vi "IKA_Eurostar60_Setup.vi"(7 "Checkbox":bool=TRUE, 8 "error in":errorcluster, 11 "COMMS":T1={"IKA_Eurostar"="COM1", "IKA"=FALSE, "Agilent"="COM1", "AGL"=FALSE}) -> (0 "error out":errorcluster)   [LabVIEW 2017]
uses:
  CRISTALIZADOR_COMM.ctl
  IKA_Eurostar60.ctl
panel:
  out "RUN":bool
  out "Par":dbl(knob) caption="Gauge" scale=0.0..10.0
  in  "Power On Button":bool
  out "PAR":dbl
  out "VELOCIDAD":dbl
  out "Velocidad":dbl(knob) caption="Gauge" scale=0.0..10.0
  out "Velocidad":dbl
  out "SETPOINT":dbl
  in  "Speed Button":bool
  in  "Giro Button":bool
  in  "Stop Button":bool
  in  "Start Button":bool
  # "Configuración rotador IKA.Euro60"
  # "asslcdms Feb2023 LV17"
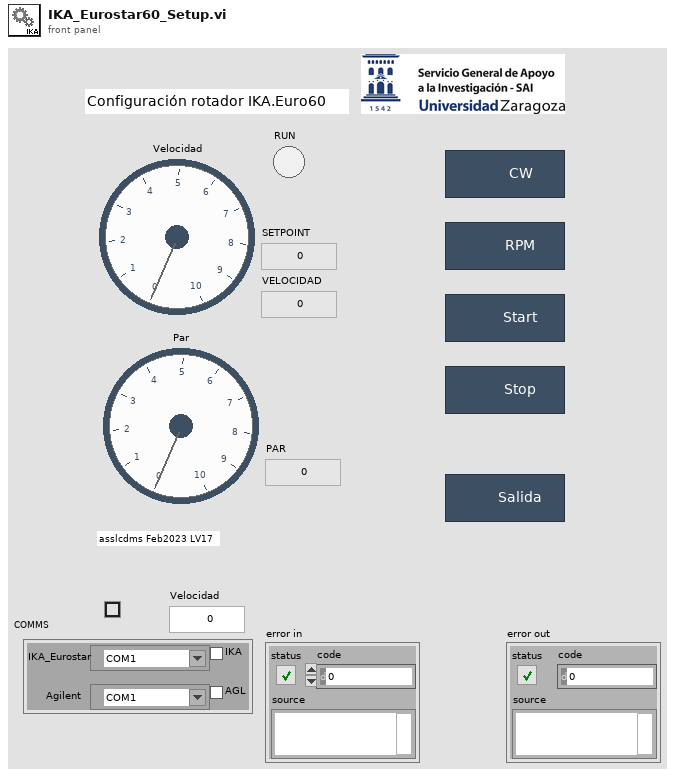
[diagram p1: front panel]
types:
  T1 = typedef "CRISTALIZADOR_COMM.ctl" = cluster{"IKA_Eurostar":refnum<visa-resource-name>, "IKA":bool, "Agilent":refnum<visa-resource-name>, "AGL":bool}
  T2 = typedef "IKA_Eurostar60.ctl" = enum16{"INICIALIZAR", "READ NOMBRE APARATO", "READ VALOR PT100", "READ VELOCIDAD ACTUAL", "READ PAR DE GIRO ACTUAL", "READ VELOCIDAD NOMINAL", "READ LIMITE PAR DE GIRO", "READ LIMITE VELOCIDAD", "READ VELOCIDAD SEGURIDAD", "SET VELOCIDAD NOMINAL", "SET LIMITE PAR DE GIRO", "SET LIMITE VELOCIDAD", "SET VELOCIDAD SEGURIDAD", "ARRANCAR MOTOR", "DETENER MOTOR", "RESET", "SET SENTIDO DE GIRO", "READ SENTIDO DE GIRO", "FINALIZAR"}
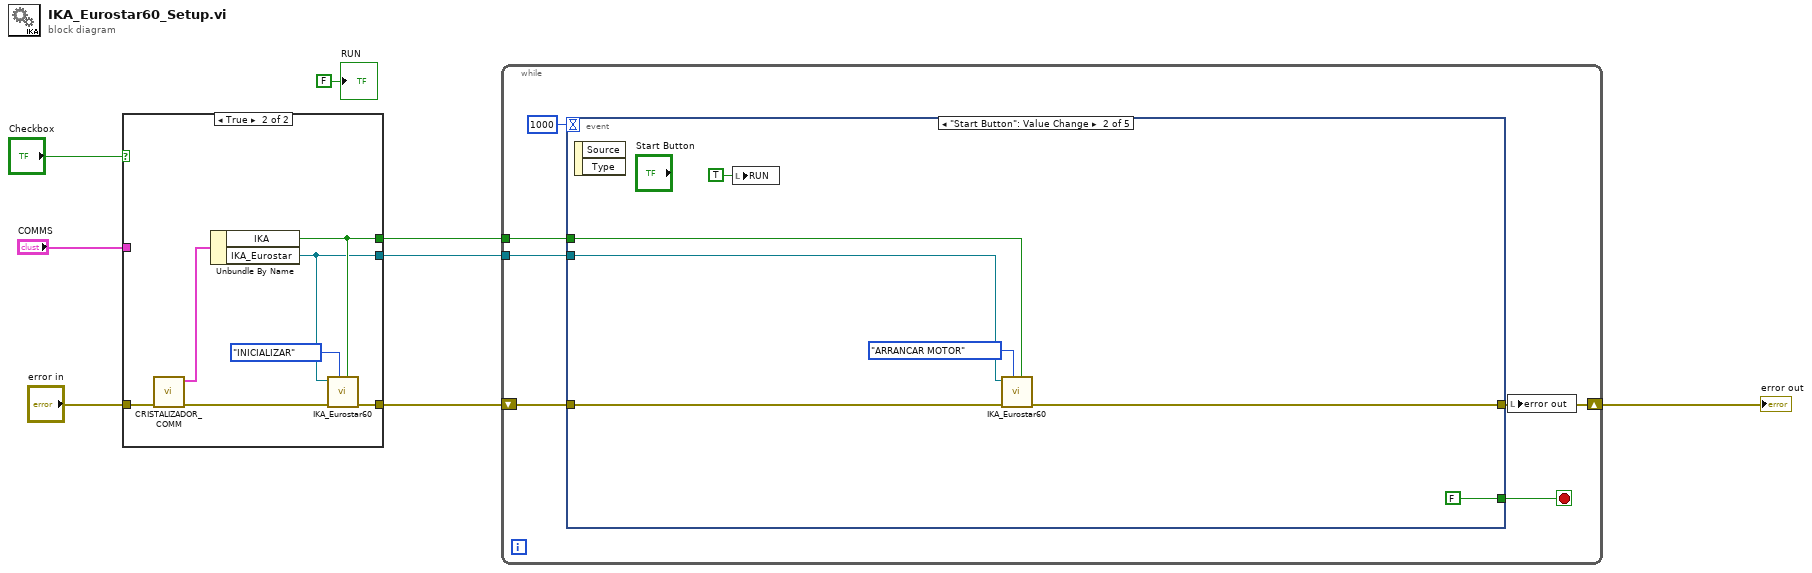
[diagram p0: block diagram]
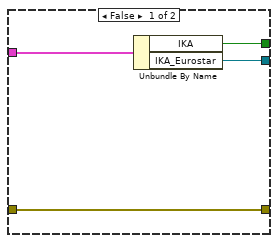
[diagram p2: hidden frame]
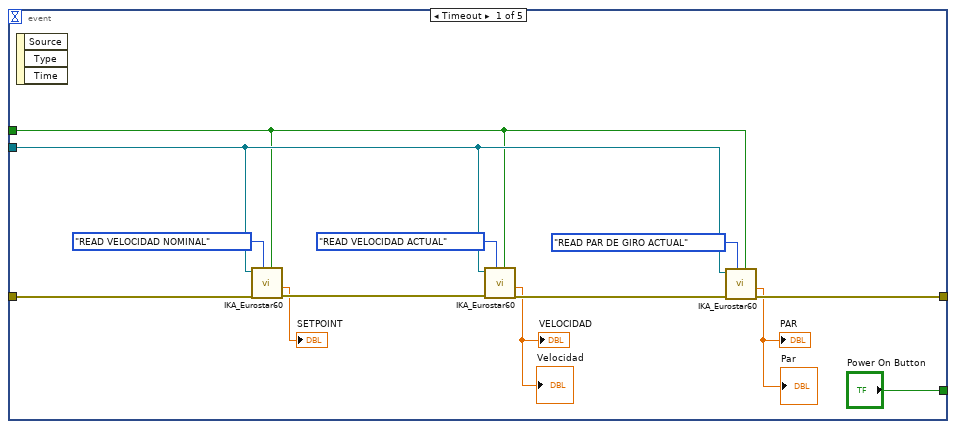
[diagram p3: hidden frame]
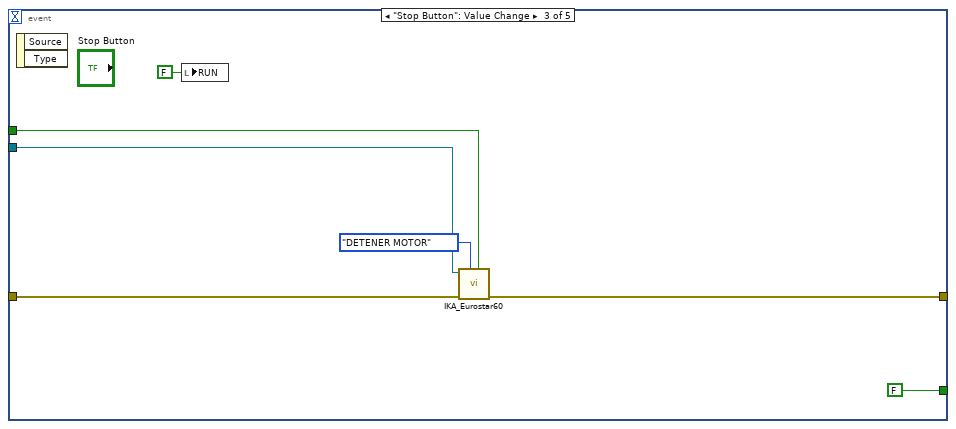
[diagram p4: hidden frame]
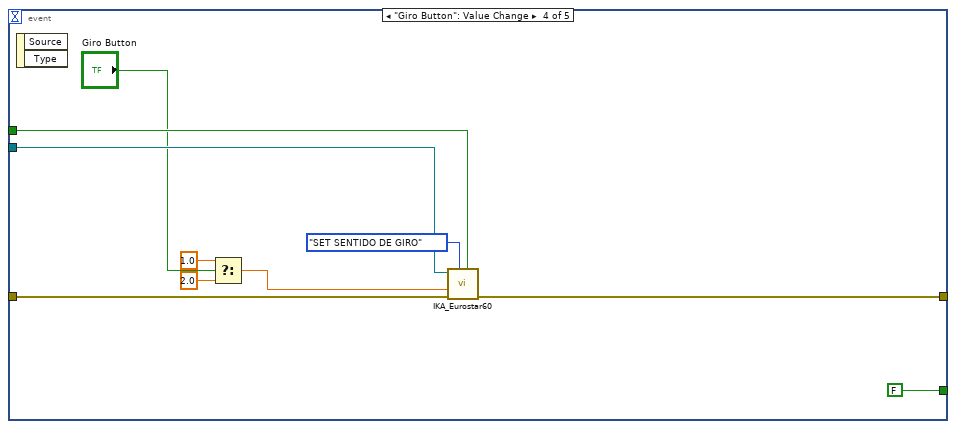
[diagram p5: hidden frame]
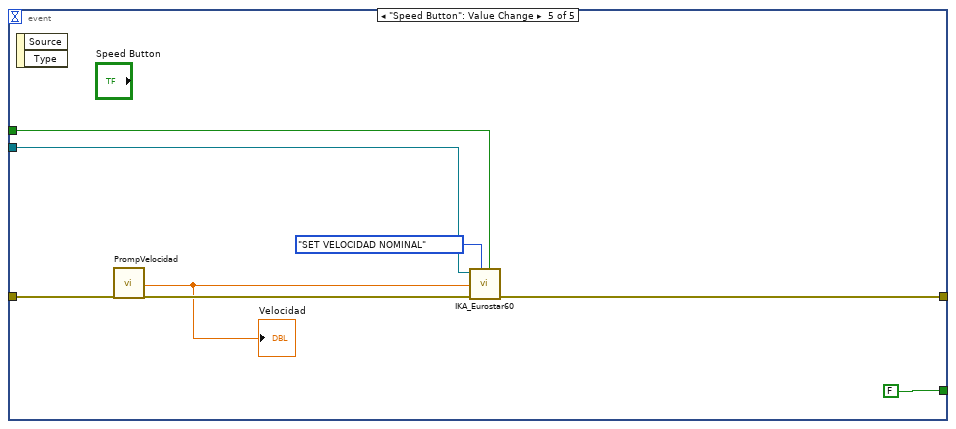
[diagram p6: hidden frame]
diagram:
  n1 = case shown="True" "Checkbox" {
    tunnel: "error in" -> [w12 w17]
    tunnel: [w12 w18] -> w6
    tunnel: "COMMS" -> [w10 _]
    tunnel: [w11 w14] -> w4
    tunnel: [w9 w13] -> w3
    frame False {
      n2 = Unbundle By Name(w10) -> ("IKA"=w11:bool, "IKA_Eurostar"=w9:refnum<visa-resource-name>)
    }
    frame True {
      n3 = call "CRISTALIZADOR_COMM.vi"("error in (no error)"=w17) -> ("error out"=w16:errorcluster, "Comunicaciones"=w15:T1)  [unwired: 8 in, 1 out]
      n4 = Unbundle By Name(w15) -> ("IKA"=w14:bool, "IKA_Eurostar"=w13:refnum<visa-resource-name>)
      n5 = call "IKA_Eurostar60.vi"("IKAenable"=w14, "Command"=IKA_Eurostar60."INICIALIZAR", "Error in"=w16, "VISA Paar mPDS2000"=w13) -> ("error out"=w18:errorcluster)  [unwired: 5 in, 2 out]
    }
  }
  n6 = while {
    tunnel: w4 -> [w25]
    tunnel: w3 -> [w24]
    shift-right: [w22] -> w8
    shift-left: w6 -> [w23]
    stop <- w20 stop-if-true
    n7 = event shown="[1] \"Start Button\": Value Change" {
      selector: _ -> [_ _ _ _ _]
      dyn-events: _ -> [_ _ _ _ _]
      timeout: 1000 -> [_ _ _ _ _]
      tunnel: w25 -> [w31 w41 w49 w59 w68]
      tunnel: w24 -> [w33 w42 w48 w58 w67]
      tunnel: [w30 w43 w50 w60 w69] -> w22
      tunnel: w23 -> [w29 w44 w51 w61 w66]
      tunnel: ["Power On Button" FALSE ("Exit Button") FALSE ("Exit Button") FALSE ("Exit Button") FALSE ("Exit Button")] -> w20
      event Timeout {
        n8 = event-data() -> ()  [unwired: 1 in, 3 out]
        n9 = call "IKA_Eurostar60.vi"("IKAenable"=w31, "Command"=IKA_Eurostar60."READ VELOCIDAD NOMINAL", "Error in"=w29, "VISA Paar mPDS2000"=w33) -> ("error out"=w37:errorcluster, "Read_parametro"=→"SETPOINT":dbl)  [unwired: 5 in, 1 out]
        n10 = call "IKA_Eurostar60.vi"("IKAenable"=w31, "Command"=IKA_Eurostar60."READ VELOCIDAD ACTUAL", "Error in"=w37, "VISA Paar mPDS2000"=w33) -> ("error out"=w38:errorcluster, "Read_parametro"=→"VELOCIDAD" →"Velocidad":dbl)  [unwired: 5 in, 1 out]
        n11 = call "IKA_Eurostar60.vi"("IKAenable"=w31, "Command"=IKA_Eurostar60."READ PAR DE GIRO ACTUAL", "Error in"=w38, "VISA Paar mPDS2000"=w33) -> ("error out"=w30:errorcluster, "Read_parametro"=→"PAR" →"Par":dbl)  [unwired: 5 in, 1 out]
      }
      event "Start Button": Value Change {
        n12 = event-data() -> ()  [unwired: 1 in, 2 out]
        n13 = local write "RUN"(TRUE ("RUN")) -> ()
        n14 = call "IKA_Eurostar60.vi"("IKAenable"=w41, "Command"=IKA_Eurostar60."ARRANCAR MOTOR", "Error in"=w44, "VISA Paar mPDS2000"=w42) -> ("error out"=w43:errorcluster)  [unwired: 5 in, 2 out]
      }
      event "Stop Button": Value Change {
        n15 = event-data() -> ()  [unwired: 1 in, 2 out]
        n16 = local write "RUN"(FALSE ("RUN")) -> ()
        n17 = call "IKA_Eurostar60.vi"("IKAenable"=w49, "Command"=IKA_Eurostar60."DETENER MOTOR", "Error in"=w51, "VISA Paar mPDS2000"=w48) -> ("error out"=w50:errorcluster)  [unwired: 5 in, 2 out]
      }
      event "Giro Button": Value Change {
        n18 = event-data() -> ()  [unwired: 1 in, 2 out]
        n19 = Select(t=1.0, s="Giro Button", f=2.0) -> (s? t:f=w54:dbl)
        n20 = call "IKA_Eurostar60.vi"("IKAenable"=w59, "Command"=IKA_Eurostar60."SET SENTIDO DE GIRO", "Error in"=w61, "Set_parametro"=w54, "VISA Paar mPDS2000"=w58) -> ("error out"=w60:errorcluster)  [unwired: 4 in, 2 out]
      }
      event "Speed Button": Value Change {
        n21 = event-data() -> ()  [unwired: 1 in, 2 out]
        n22 = call "PrompVelocidad.vi"("error in (no error)"=w66) -> ("Velocidad"=w64:dbl, "error out"=w65:errorcluster)  [unwired: 16 in, 1 out]
        "Velocidad" <- w64
        n23 = call "IKA_Eurostar60.vi"("IKAenable"=w68, "Command"=IKA_Eurostar60."SET VELOCIDAD NOMINAL", "Error in"=w65, "Set_parametro"=w64, "VISA Paar mPDS2000"=w67) -> ("error out"=w69:errorcluster)  [unwired: 4 in, 2 out]
      }
    }
    n24 = local write "error out"(w22) -> ()
  }
  "error out" <- w8
  "RUN" <- FALSE ("RUN")
